vi "Gear Delivery SS Implem.vi"(11 "Gear Delivery Commands In":T1) -> (3 "Gear Delivery Actuators Out":T2={"Gear Release"=enum."Reverse", "Gear Intake"=enum."Off", "Gear Chute"=enum."Off"})   [LabVIEW 2016]
uses:
  Gear Delivery Actuator Out.ctl
  Gear Delivery Commands.ctl
  <vilib>/Rock Robotics/WPI/Solenoid/WPI_SolenoidValue.ctl
  Gear Delivery Logging Values.vi
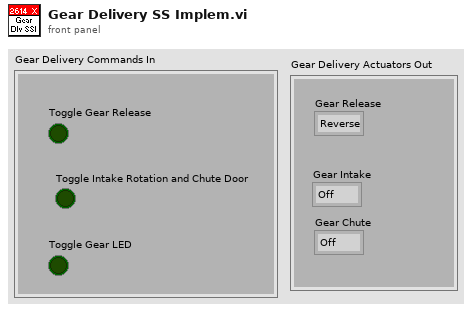
[diagram p1: front panel]
types:
  T1 = typedef "Gear Delivery Commands.ctl" = cluster{"Toggle Gear Release":bool, "Toggle Intake Rotation and Chute Door":bool, "Toggle Gear LED":bool}
  T2 = typedef "Gear Delivery Actuator Out.ctl" = cluster{"Gear Release":enum16{"Off", "On", "Forward", "Reverse"}, "Gear Intake":enum16{"Off", "On", "Forward", "Reverse"}, "Gear Chute":enum16{"Off", "On", "Forward", "Reverse"}}
  T3 = typedef "WPI_SolenoidValue.ctl" = enum16{"Off", "On", "Forward", "Reverse"}
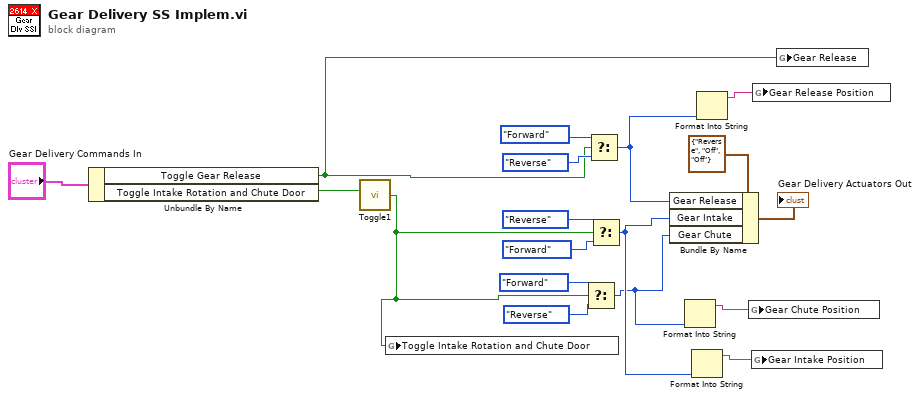
[diagram p0: block diagram]
diagram:
  n1 = Unbundle By Name("Gear Delivery Commands In") -> ("Toggle Gear Release"=w5:bool, "Toggle Intake Rotation and Chute Door"=w10:bool)
  n2 = call "Toggle1.vi"("Boolean"=w10) -> ("Driver Switch 2"=w3:bool)
  n3 = global write "Gear Delivery Logging Values.vi" "Toggle Intake Rotation and Chute Door"(w3) -> ()
  n4 = Select(t=WPI_SolenoidValue."Forward" ("Value"), s=w3, f=WPI_SolenoidValue."Reverse" ("Value")) -> (s? t:f=w6:T3)
  n5 = Select(t=WPI_SolenoidValue."Forward" ("Value"), s=w5, f=WPI_SolenoidValue."Reverse" ("Value")) -> (s? t:f=w11:T3)
  n6 = Select(t=WPI_SolenoidValue."Reverse" ("Value"), s=w3, f=WPI_SolenoidValue."Forward" ("Value")) -> (s? t:f=w9:T3)
  n7 = Bundle By Name(cluster=T2 {"Gear Release"=enum."Reverse", "Gear Intake"=enum."Off", "Gear Chute"=enum."Off"} ("Gear Delivery Actuators Out 2"), "Gear Release"=w11, "Gear Intake"=w9, "Gear Chute"=w6) -> (→"Gear Delivery Actuators Out":T2)
  n8 = Format Into String(w6) -> (resulting string=w1:string)  [unwired: 3 in, 1 out]
  n9 = Format Into String(w9) -> (resulting string=w2:string)  [unwired: 3 in, 1 out]
  n10 = Format Into String(w11) -> (resulting string=w4:string)  [unwired: 3 in, 1 out]
  n11 = global write "Gear Delivery Logging Values.vi" "Gear Chute Position"(w1) -> ()
  n12 = global write "Gear Delivery Logging Values.vi" "Gear Intake Position"(w2) -> ()
  n13 = global write "Gear Delivery Logging Values.vi" "Gear Release Position"(w4) -> ()
  n14 = global write "Gear Delivery Logging Values.vi" "Gear Release"(w5) -> ()
